vi "LineTrackerMovement.vi"(9 "Right Line Sensor":bool, 10 "Center Line Sensor":bool, 11 "Left Line Sensor":bool) -> (2 "Right motor":dbl, 3 "Left Motor":dbl)   [LabVIEW 2018]
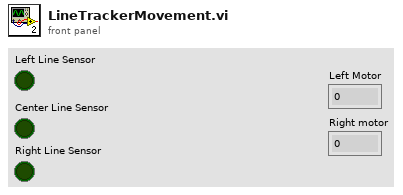
[diagram p1: front panel]
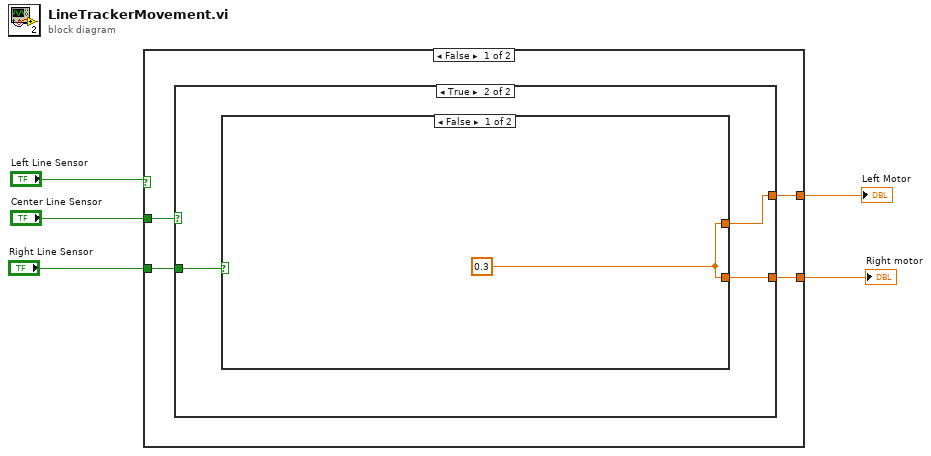
[diagram p0: block diagram]
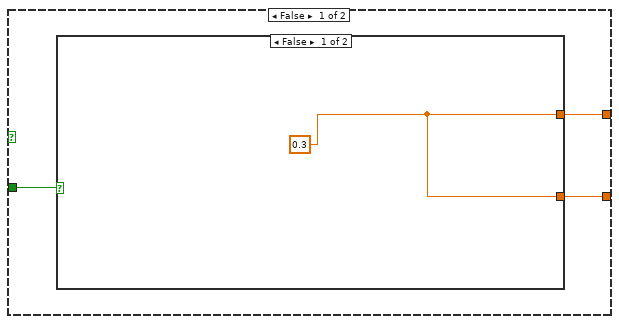
[diagram p2: hidden frame]
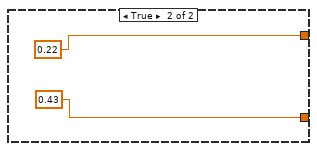
[diagram p3: hidden frame]
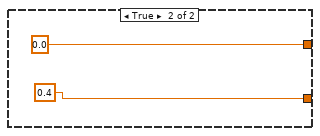
[diagram p4: hidden frame]
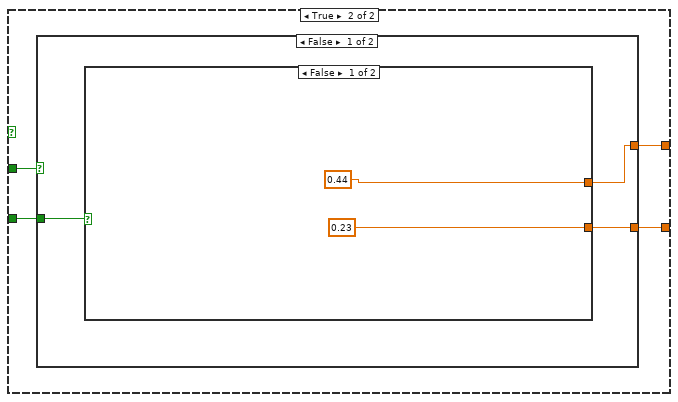
[diagram p5: hidden frame]
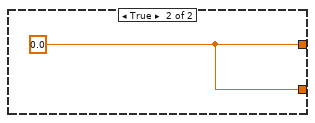
[diagram p6: hidden frame]
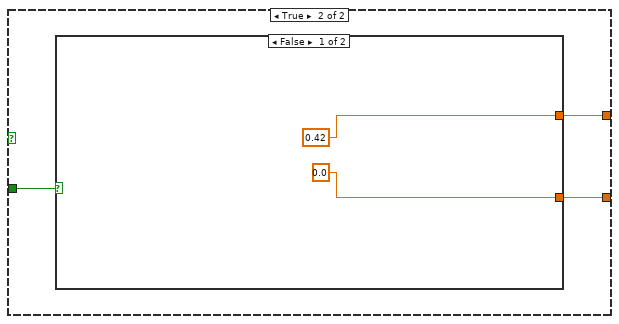
[diagram p7: hidden frame]
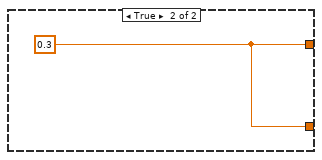
[diagram p8: hidden frame]
diagram:
  n1 = case shown="False" "Left Line Sensor" {
    tunnel: "Center Line Sensor" -> [w9 w25]
    tunnel: "Right Line Sensor" -> [w8 w24]
    tunnel: [w7 w23] -> w2
    tunnel: [w6 w22] -> w1
    frame False {
      n2 = case shown="True" w9 {
        tunnel: w8 -> [w12 w18]
        tunnel: [w11 w16] -> w7
        tunnel: [w10 w17] -> w6
        frame False {
          n3 = case shown="False" w12 {
            tunnel: [w13 0.22 ("Left Motor")] -> w11
            tunnel: [w13 0.43 ("Left Motor")] -> w10
            frame False {
              w13 = 0.3 ("Left Motor")
            }
            frame True {
            }
          }
        }
        frame True {
          n4 = case shown="False" w18 {
            tunnel: [w19 0.4 ("Left Motor")] -> w17
            tunnel: [w19 0.0 ("Left Motor")] -> w16
            frame False {
              w19 = 0.3 ("Left Motor")
            }
            frame True {
            }
          }
        }
      }
    }
    frame True {
      n5 = case shown="False" w25 {
        tunnel: w24 -> [w28 w34]
        tunnel: [w27 w33] -> w23
        tunnel: [w26 w32] -> w22
        frame False {
          n6 = case shown="False" w28 {
            tunnel: [0.44 ("Left Motor") w31] -> w27
            tunnel: [0.23 ("Left Motor") w31] -> w26
            frame False {
            }
            frame True {
              w31 = 0.0 ("Left Motor")
            }
          }
        }
        frame True {
          n7 = case shown="False" w34 {
            tunnel: [0.42 ("Left Motor") w37] -> w33
            tunnel: [0.0 ("Left Motor") w37] -> w32
            frame False {
            }
            frame True {
              w37 = 0.3 ("Left Motor")
            }
          }
        }
      }
    }
  }
  "Left Motor" <- w2
  "Right motor" <- w1
